vi "Drive Straight PID.vi"(6 "Force? (F)":bool, 7 "Wait for Completion? (F)":bool, 8 "error in":errorcluster, 10 "angle offset (0)":dbl, 11 "Distance (in)":dbl) -> (0 "error out":errorcluster)   [LabVIEW 2016, in "Drive System.lvlib"]
uses:
  Drive System.lvlib
  Private/DriveCmd.ctl
  Private/DriveCmdList.ctl
  Private/Varient Cmd Types/Drive PID CMD.ctl
panel:
  in  "Timeout ms (-1)":i32=-1
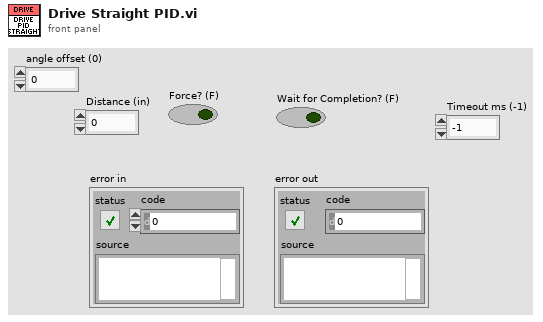
[diagram p1: front panel]
types:
  T1 = typedef "Drive System.lvlib/Drive PID CMD.ctl" = cluster{"distance":dbl, "angle offset (0)":dbl}
  T2 = typedef "Drive System.lvlib/DriveCmd.ctl" = cluster{"cmd":T3, "data":variant, "Force? (F)":bool, "Lock":string}
  T3 = typedef "Drive System.lvlib/DriveCmdList.ctl" = enum16{"Idle", "Cleanup", "Drive For Time", "Follow Path Speed Control", "Follow Path", "Drive Tank", "Drive Straight PID", "Drive Angle Mag", "Drive Arcade", "Drive Ref", "Unlock", "Lock"}
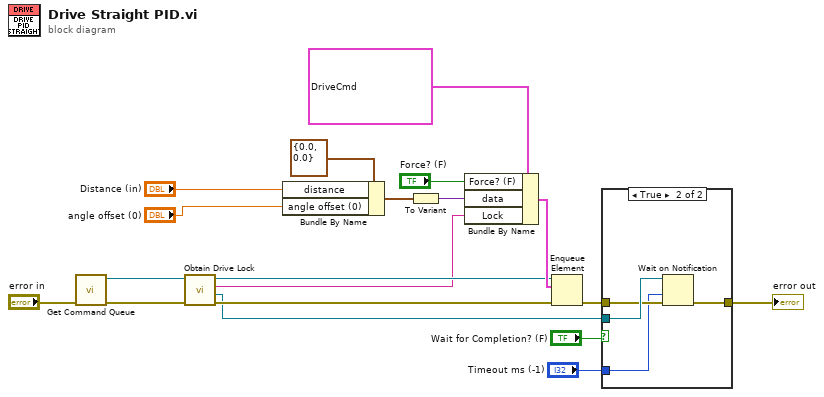
[diagram p0: block diagram]
diagram:
  n1 = call "Get Command Queue.vi"("error in (no error)"="error in") -> ("error out"=w19:errorcluster, "Queue out"=w18:refnum<queue>)  [unwired: 9 in]
  n2 = call "Obtain Drive Lock.vi"("error in"=w19, "Queue in"=w18) -> ("error out"=w12:errorcluster, "notifier out"=w7:refnum<notifier>, "Lock"=w10:string, "queue out"=w11:refnum<queue>)  [unwired: 6 in]
  n3 = Bundle By Name(cluster=T1 {"distance"=0.0, "angle offset (0)"=0.0} ("Cluster"), "distance"="Distance (in)", "angle offset (0)"="angle offset (0)") -> (w3:T1)
  n4 = To Variant(anything=w3) -> (Variant=w15:variant)
  n5 = Bundle By Name(cluster=T2 {"cmd"=enum."Drive Straight PID", "data"=variant, "Force? (F)"=FALSE, "Lock"=""} ("element"), "Force? (F)"="Force? (F)", "data"=w15, "Lock"=w10) -> (w16:T2)
  n6 = Enqueue Element(queue=w11, element=w16, error in (no error)=w12) -> (error out=w8:errorcluster)  [unwired: 1 in, 2 out]
  n7 = case shown="True" "Wait for Completion? (F)" {
    tunnel: w8 -> [w20 w23]
    tunnel: w7 -> [_ w24]
    tunnel: [w20 w22] -> w6
    tunnel: "Timeout ms (-1)" -> [_ w21]
    frame False {
    }
    frame True {
      n8 = Wait on Notification(notifier=w24, timeout in ms (-1)=w21, error in (no error)=w23) -> (error out=w22:errorcluster)  [unwired: 1 in, 3 out]
    }
  }
  "error out" <- w6
